vi "finalize cipher.vi"(8 "error in":errorcluster, 11 "lvlibcrypto cipher in":refnum<class "lvlibcrypto cipher.lvclass">) -> (0 "error out":errorcluster, 2 "data out":string, 3 "lvlibcrypto cipher out":refnum<class "lvlibcrypto cipher.lvclass">)   [LabVIEW 2016, in "lvlibcrypto cipher.lvclass"]
uses:
  lvlibcrypto cipher.lvclass
  lvlibcrypto cipher.lvclass/lvlibcrypto cipher.ctl
  lv tls dll.lvlib
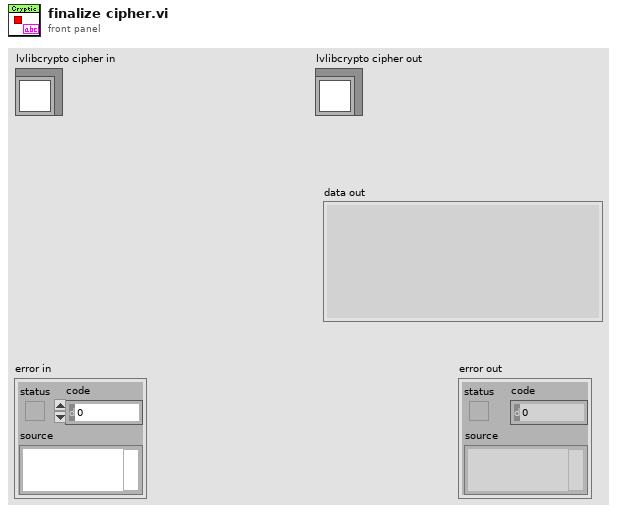
[diagram p1: front panel]
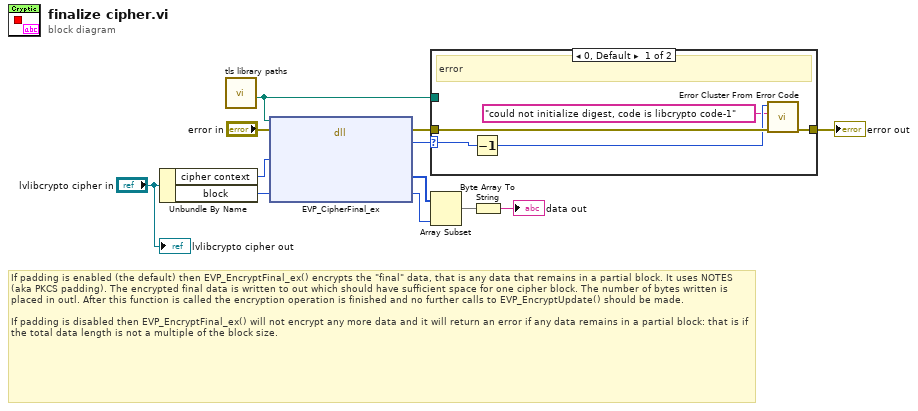
[diagram p0: block diagram]
diagram:
  # "If padding is enabled (the default) then EVP_EncryptFinal_ex() encrypts the \"final\" data, that is any data that remains in a partial block. It uses NOTES (aka PKCS padding). The encrypted final data is written to out which should have sufficient space for one cipher block. The number of bytes written is placed in outl. After this function is called the encryption operation is finished and no further calls to EVP_EncryptUpdate() should be made.\n\nIf padding is disabled then EVP_EncryptFinal_ex() will not encrypt any more data and it will return an error if any data remains in a partial block: that is if the total data length is not a multiple of the block size."
  n1 = Unbundle By Name("lvlibcrypto cipher in") -> ("cipher context"=w8:u64, "block"=w2:i32)
  n2 = call "tls library paths.vi"() -> ("libcrypto"=w9:path)  [unwired: 8 in, 3 out]
  n3 = dll-call lib="C:/Users/IEUser/Desktop/tlssimple/libcrypto-41.dll" fn="EVP_CipherFinal_ex"(path in=w9, error in="error in", "context"=w8, "length"=w2) -> (error out=w11:errorcluster, "ret"=w12:i32, "dataout"=w7:u8[], "length"=w6:i32)  [unwired: 3 in, 1 out]
  n4 = case shown="0, Default" w12 {
    selector: w12 -> [w15 _]
    tunnel: [w16 w18] -> w10
    tunnel: w11 -> [w17 w18]
    tunnel: w9 -> [_ _]
    frame 0, Default {
      # "error"
      n5 = Decrement(x=w15) -> (x-1=w14:i32)
      n6 = call <vilib>:"Error Cluster From Error Code.vi"("error in (no error)"=w17, "error message (\"\")"="could not initialize digest, code is libcrypto code-1" ("error message (\"\")"), "error code (0)"=w14) -> ("error out"=w16:errorcluster)  [unwired: 6 in]
    }
    frame 1 {
      # "success"
    }
  }
  "error out" <- w10
  n7 = Array Subset(array=w7, length=w6) -> (w5:u8[])  [unwired: 1 in]
  n8 = Byte Array To String(unsigned byte array=w5) -> (string=→"data out":string)
  "lvlibcrypto cipher out" <- "lvlibcrypto cipher in"
